vi "Diagnostics Get Data and Subfunction.vi"(3 "data in":u8[](array[numeric])) -> (0 "subfunction":u16, 1 "data out":u8[](array[numeric]))   [LabVIEW 2021, in "Modbus Library.lvlib" / "Master Function Definition.lvclass"]
uses:
  Master Function Definition.lvclass
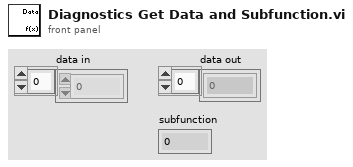
[diagram p1: front panel]
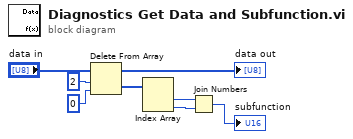
[diagram p0: block diagram]
diagram:
  n1 = Delete From Array(array="data in", length=2, index=0) -> (deleted portion=w7:u8[], array with subset deleted=→"data out":u8[])
  n2 = Index Array(array=w7) -> (element #1=w3:u8, element #2=w2:u8)  [unwired: 2 in]
  n3 = Join Numbers(hi=w3, lo=w2) -> ((hi.lo)=→"subfunction":u16)
